vi "Verify Set and Get Accessors for DSF Configuration.vi"(6 ".NET Refnum":refnum<k24>, 8 "error in":errorcluster, 10 "version":cluster{"major":u32, "minor":u32, "update":u32}={"major"=1, "minor"=0, "update"=0}, 11 "Set and Get Config Options Test in":refnum<class "Set and Get Config Options Test.lvclass">) -> (0 "error out":errorcluster, 3 "Set and Get Config Options Test out":refnum<class "Set and Get Config Options Test.lvclass">)   [LabVIEW 2020, in "Set and Get Config Options Test.lvclass"]
uses:
  Set and Get Config Options Test.lvclass
  Scripting API/Data Sharing Framework Custom Device Scripting.lvlib
  Shared/DSF Shared.lvlib
  NationalInstruments.VeriStand.SystemDefinitionAPI
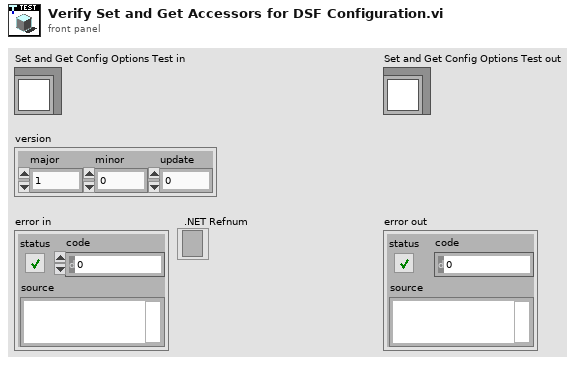
[diagram p1: front panel]
types:
  T1 = typedef "Custom Device API.lvlib/Custom Device Item Ref.ctl" = u64
  T2 = typedef "DSF Core.lvlibp/Framework.lvclass/Framework Options.ctl" = cluster{"FIFO Options":T3, "Thread Options":T4, "Plugin Options":T5, "Performance Options":T6, "Data Server Options":T7}
  T3 = typedef "DSF Core.lvlibp/Framework.lvclass/DSF FIFO Options.ctl" = cluster{"Infinite Timeouts":bool}
  T4 = typedef "DSF Core.lvlibp/Thread.lvclass/Thread Options.ctl" = cluster{"Show FP On Call":bool, "Close FP After Call":bool, "Allow Debugging":bool}
  T5 = typedef "DSF Core.lvlibp/Framework.lvclass/DSF Plugin Options.ctl" = cluster{"Default Components":bool}
  T6 = typedef "DSF Core.lvlibp/DSF Performance Options.ctl" = cluster{"Measure Period":bool, "Measure Rx/Tx Duration":bool}
  T7 = typedef "DSF Core.lvlibp/Framework.lvclass/Data Server Options.ctl" = cluster{"Enable Data Server":bool, "Period":u32}
  T8 = cluster{"measure period?":bool, "measure Rx/Tx duration?":bool}
  T9 = cluster{"enable data server":bool, "data server frequency (Hz)":dbl, "enable data server":bool}
  T10 = cluster{"data server enabled?":bool, "data server frequency (Hz)":dbl, "launch data viewer?":bool}
  T11 = cluster{"debug?":bool, "infinite FIFO timeouts?":bool}
  T12 = cluster{"show error dialog":bool, "show error dialog":bool}
  T13 = cluster{"show error dialog?":bool, "show threads?":bool}
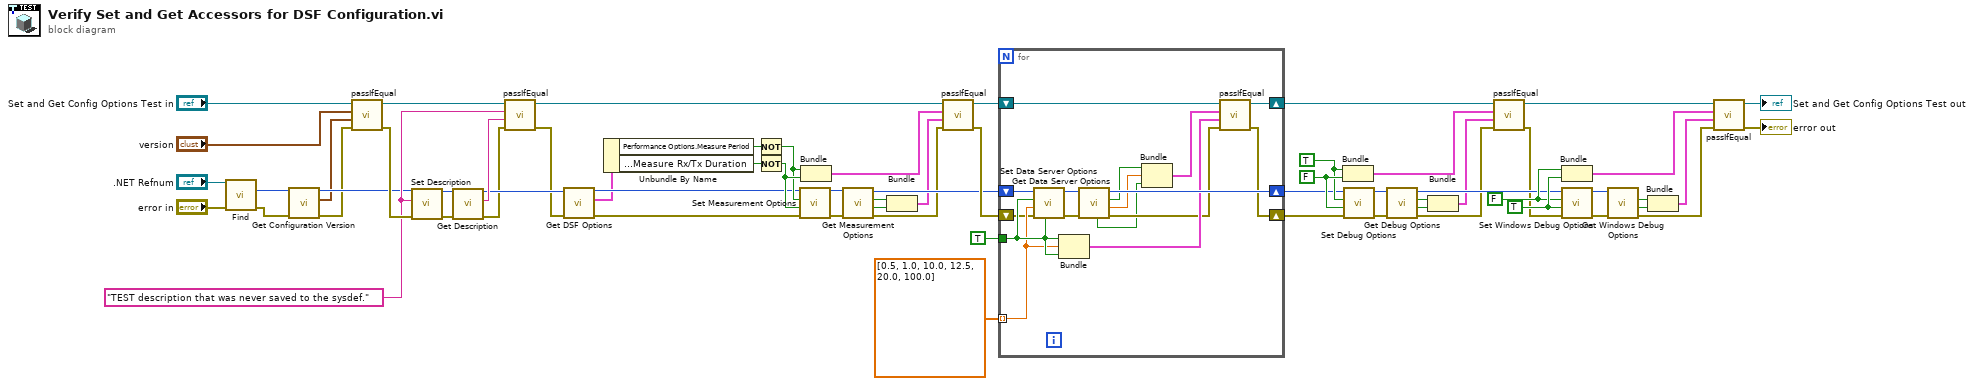
[diagram p0: block diagram]
diagram:
  w1 = dbl[] [0.5, 1.0, 10.0, 12.5, 20.0, 100.0] items=["0.5 Hz"=0.5, "1.0 Hz"=1.0, "2.0 Hz"=2.0, "2.5 Hz"=2.5, "4.0 Hz"=4.0, "5.0 Hz"=5.0, "8.0 Hz"=8.0, "10.0 Hz"=10.0, "12.5 Hz"=12.5, "20.0 Hz"=20.0, "25.0 Hz"=25.0, "40.0 Hz"=40.0, "50.0 Hz"=50.0, "100.0 Hz"=100.0]
  w57 = TRUE ("show error dialog")
  w56 = FALSE ("show error dialog")
  w44 = FALSE ("debug")
  w43 = TRUE ("debug")
  w13 = "TEST description that was never saved to the sysdef." ("description")
  n1 = call "Find.vi"("error in"="error in", "target in"=".NET Refnum") -> ("error out"=w6:errorcluster, "data sharing framework custom device"=w5:T1)  [unwired: 6 in, 2 out]
  n2 = call "Get Configuration Version.vi"("error in"=w6, "data sharing framework custom device in"=w5) -> ("error out"=w9:errorcluster, "version"=w8:cluster{"major":u32, "minor":u32, "update":u32}, "data sharing framework custom device out"=w10:T1)  [unwired: 6 in, 1 out]
  n3 = call-dynamic "passIfEqual.vi"("error in (no error)"=w9, "y"=w8, "x"="version", "TestCase in"="Set and Get Config Options Test in") -> ("error out"=w14:errorcluster, "TestCase out"=w12:refnum<class "Set and Get Config Options Test.lvclass">)  [unwired: 6 in]
  n4 = call "Set Description.vi"("error in"=w14, "description"=w13, "data sharing framework custom device in"=w10) -> ("error out"=w15:errorcluster, "data sharing framework custom deviceout"=w11:T1)  [unwired: 7 in]
  n5 = call "Get Description.vi"("error in"=w15, "data sharing framework custom device in"=w11) -> ("error out"=w16:errorcluster, "description"=w19:string, "data sharing framework custom deviceout"=w18:T1)  [unwired: 7 in]
  n6 = call-dynamic "passIfEqual.vi"("error in (no error)"=w16, "y"=w19, "x"=w13, "TestCase in"=w12) -> ("error out"=w17:errorcluster, "TestCase out"=w34:refnum<class "Set and Get Config Options Test.lvclass">)  [unwired: 6 in]
  n7 = call "Get DSF Options.vi"("error in (no error)"=w17, "Item Ref in"=w18) -> ("error out"=w24:errorcluster, "options"=w20:T2, "Item Ref out"=w23:T1)  [unwired: 7 in]
  n8 = Unbundle By Name(w20) -> ("Performance Options.Measure Period"=w21:bool, "Performance Options.Measure Rx/Tx Duration"=w22:bool)
  n9 = Not(x=w21) -> (.not. x?=w27:bool)
  n10 = Not(x=w22) -> (.not. x?=w28:bool)
  n11 = call "Set Measurement Options.vi"("error in"=w24, "measure Rx/Tx duration"=w28, "measure period"=w27, "data sharing framework custom device in"=w23) -> ("error out"=w26:errorcluster, "data sharing framework custom device out"=w25:T1)  [unwired: 6 in]
  n12 = Bundle(w27, w28) -> (w32:cluster{bool, bool})  [unwired: 1 in]
  n13 = call "Get Measurement Options.vi"("error in"=w26, "data sharing framework custom device in"=w25) -> ("error out"=w33:errorcluster, "measure Rx/Tx duration?"=w30:bool, "measure period?"=w29:bool, "data sharing framework custom device out"=w35:T1)  [unwired: 6 in]
  n14 = Bundle("measure period?"=w29, "measure Rx/Tx duration?"=w30) -> (w31:T8)  [unwired: 1 in]
  n15 = call-dynamic "passIfEqual.vi"("error in (no error)"=w33, "y"=w31, "x"=w32, "TestCase in"=w34) -> ("error out"=w36:errorcluster, "TestCase out"=w38:refnum<class "Set and Get Config Options Test.lvclass">)  [unwired: 6 in]
  n16 = for {
    tunnel: TRUE ("enable data server") -> [w70]
    tunnel: w1 -> [w69] mode=indexing
    shift-right: [w80] -> w48
    shift-left: w38 -> [w74]
    shift-right: [w78] -> w39
    shift-left: w36 -> [w67]
    shift-right: [w79] -> w40
    shift-left: w35 -> [w65]
    n17 = call "Set Data Server Options.vi"("launch data viewer"=w70, "error in"=w67, "data server frequency (Hz)"=w69, "enable data server"=w70, "data sharing framework custom device in"=w65) -> ("error out"=w68:errorcluster, "data sharing framework custom device out"=w66:T1)  [unwired: 4 in, 1 out]
    n18 = Bundle("enable data server"=w70, "data server frequency (Hz)"=w69, "enable data server"=w70) -> (w76:T9)  [unwired: 1 in]
    n19 = call "Get Data Server Options.vi"("error in"=w68, "data sharing framework custom device in"=w66) -> ("error out"=w75:errorcluster, "data server frequency (Hz)"=w72:dbl, "data server enabled?"=w71:bool, "data sharing framework custom device out"=w79:T1, "launch data viewer?"=w73:bool)  [unwired: 5 in]
    n20 = Bundle("data server enabled?"=w71, "data server frequency (Hz)"=w72, "launch data viewer?"=w73) -> (w77:T10)  [unwired: 1 in]
    n21 = call-dynamic "passIfEqual.vi"("error in (no error)"=w75, "y"=w76, "x"=w77, "TestCase in"=w74) -> ("error out"=w78:errorcluster, "TestCase out"=w80:refnum<class "Set and Get Config Options Test.lvclass">)  [unwired: 6 in]
  }
  n22 = Bundle("debug"=w43, "debug"=w44) -> (w49:cluster{"debug":bool, "debug":bool})  [unwired: 1 in]
  n23 = call "Set Debug Options.vi"("error in"=w39, "infinite FIFO timeouts"=w44, "debug"=w43, "data sharing framework custom device in"=w40) -> ("error out"=w41:errorcluster, "data sharing framework custom device out"=w42:T1)  [unwired: 6 in]
  n24 = call "Get Debug Options.vi"("error in"=w41, "data sharing framework custom device in"=w42) -> ("error out"=w47:errorcluster, "infinite FIFO timeouts?"=w46:bool, "debug?"=w45:bool, "data sharing framework custom device out"=w54:T1)  [unwired: 6 in]
  n25 = Bundle("debug?"=w45, "infinite FIFO timeouts?"=w46) -> (w50:T11)  [unwired: 1 in]
  n26 = call-dynamic "passIfEqual.vi"("error in (no error)"=w47, "y"=w50, "x"=w49, "TestCase in"=w48) -> ("error out"=w53:errorcluster, "TestCase out"=w59:refnum<class "Set and Get Config Options Test.lvclass">)  [unwired: 6 in]
  n27 = Bundle("show error dialog"=w56, "show error dialog"=w57) -> (w52:T12)  [unwired: 1 in]
  n28 = call "Set Windows Debug Options.vi"("error in"=w53, "show threads"=w57, "show error dialog"=w56, "data sharing framework custom device in"=w54) -> ("error out"=w58:errorcluster, "data sharing framework custom device out"=w55:T1)  [unwired: 6 in]
  n29 = call "Get Windows Debug Options.vi"("error in"=w58, "data sharing framework custom device in"=w55) -> ("error out"=w62:errorcluster, "show threads?"=w61:bool, "show error dialog?"=w60:bool)  [unwired: 6 in, 1 out]
  n30 = Bundle("show error dialog?"=w60, "show threads?"=w61) -> (w51:T13)  [unwired: 1 in]
  n31 = call-dynamic "passIfEqual.vi"("error in (no error)"=w62, "y"=w51, "x"=w52, "TestCase in"=w59) -> ("error out"=→"error out":errorcluster, "TestCase out"=→"Set and Get Config Options Test out":refnum<class "Set and Get Config Options Test.lvclass">)  [unwired: 6 in]
